vi "test_0217.vi"   [LabVIEW 2019]
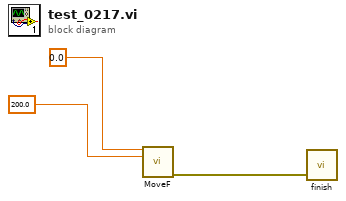
[diagram p0: block diagram]
diagram:
  n1 = call "MoveF.vi"("X"=0.0, "Y"=200.0) -> ("error out"=w3:errorcluster)  [unwired: 13 in]
  n2 = call "finish.vi"("Error/Flow In"=w3) -> ()  [unwired: 11 in]
